vi "kalman predict step multi tick interval.vi"(7 "v-feedback":bool, 10 "state in":T1) -> (2 "state out":T1)   [LabVIEW 2010]
uses:
  integrating single axis kalman state.ctl
  <vilib>/rvi/FXPMathLib/FxpMul/XNode/nifxpmath_Multiplier.xnode
  <vilib>/rvi/FXPMathLib/FxpMul/subVIs/nifxpmath_Mul_SimConfig.ctl
  <vilib>/fxp/LVFixedPointQuantizationPolicyTypeDef.ctl
  <vilib>/fxp/LVFixedPointOverflowPolicyTypeDef.ctl
  <vilib>/rvi/FXPMathLib/FxpAdd/XNode/nifxpmath_Add.xnode
  <vilib>/rvi/FXPMathLib/FxpAdd/subVIs/nifxpmath_Add_SimConfig.ctl
  <vilib>/rvi/FXPMathLib/FxpInterpret/XNode/nifxpmath_Interpret.xnode
  <vilib>/rvi/FXPMathLib/FxpMul/simVIs/DllFxpMulTemp_sub.vi
  <vilib>/rvi/FXPMathLib/FxpAdd/simVIs/DllFxpAddTemp_sub.vi
panel:
  in  "elapsed time (ticks)":u32
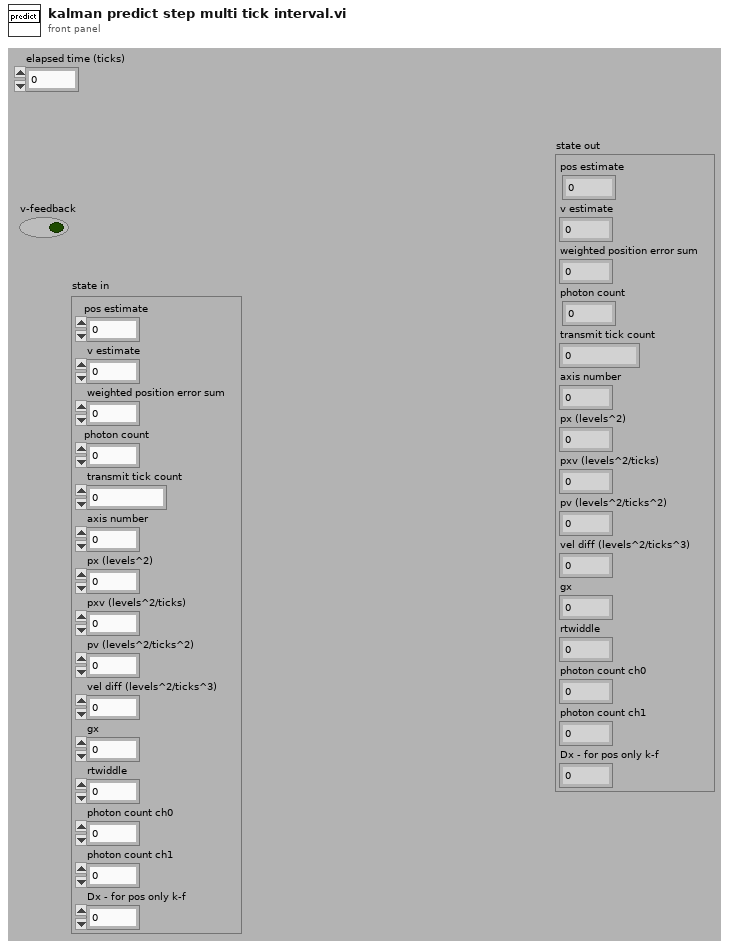
[diagram p1: front panel]
types:
  T1 = typedef "integrating single axis kalman state.ctl" = cluster{"pos estimate":fxp<+/-,32,16>, "v estimate":fxp<+/-,16,0>, "weighted position error sum":fxp<+/-,32,32>, "photon count":u32, "transmit tick count":u32, "axis number":u8, "px (levels^2)":fxp<+,32,19>, "pxv (levels^2/ticks)":fxp<+,32,2>, "pv (levels^2/ticks^2)":fxp<+,32,-14>, "vel diff (levels^2/ticks^3)":fxp<+,24,-22>, "gx":fxp<+,16,8>, "rtwiddle":fxp<+,16,26>, "photon count ch0":u32, "photon count ch1":u32, "Dx - for pos only k-f":fxp<+,32,19>}
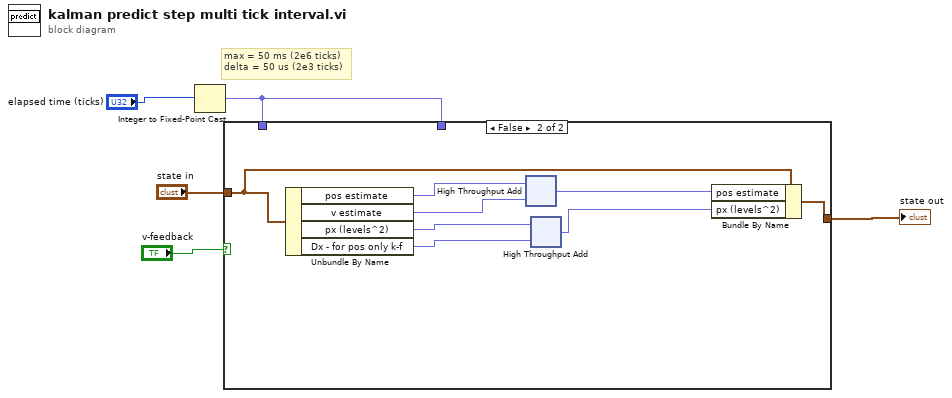
[diagram p0: block diagram]
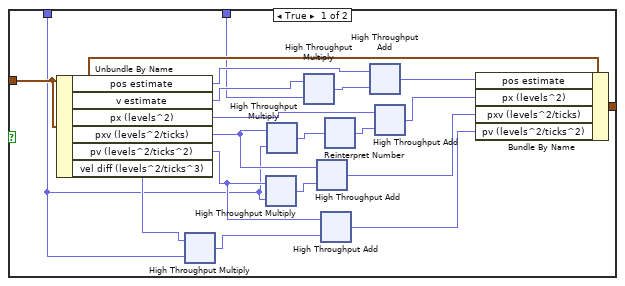
[diagram p2: hidden frame]
diagram:
  # "max = 50 ms (2e6 ticks)\ndelta = 50 us (2e3 ticks)"
  n1 = Integer to Fixed-Point Cast(integer="elapsed time (ticks)") -> (fixed-point=w1:fxp<+,10,21>)  [unwired: 1 in]
  n2 = case shown="False" "v-feedback" {
    tunnel: "state in" -> [w22 w275]
    tunnel: [w18 w273] -> w4
    tunnel: w1 -> [w14 _]
    tunnel: w1 -> [w7 _]
    frame True {
      n3 = Unbundle By Name(w22) -> ("pos estimate"=w17:fxp<+/-,32,16>, "v estimate"=w15:fxp<+/-,16,0>, "px (levels^2)"=w24:fxp<+,32,19>, "pxv (levels^2/ticks)"=w8:fxp<+,32,2>, "pv (levels^2/ticks^2)"=w10:fxp<+,32,-14>, "vel diff (levels^2/ticks^3)"=w12:fxp<+,24,-22>)
      n4 = xnode "High Throughput Multiply"("x"=w12, "y"=w7) -> ("x*y"=w11:fxp<+,16,-14>)
      n5 = xnode "High Throughput Multiply"("x"=w10, "y"=w7) -> ("x*y"=w9:fxp<+,16,2>)
      n6 = xnode "High Throughput Multiply"("x"=w8, "y"=w7) -> ("x*y"=w6:fxp<+,16,18>)
      n7 = xnode "High Throughput Multiply"("x"=w15, "y"=w14) -> ("x*y"=w13:fxp<+/-,16,15>)
      n8 = xnode "High Throughput Add"("x"=w8, "y"=w9) -> ("x+y"=w20:fxp<+,32,2>)
      n9 = xnode "High Throughput Add"("x"=w10, "y"=w11) -> ("x+y"=w19:fxp<+,32,-14>)
      n10 = xnode "Reinterpret Number"("x"=w6) -> ("y"=w23:fxp<+,16,19>)
      n11 = xnode "High Throughput Add"("x"=w17, "y"=w13) -> ("x+y"=w16:fxp<+/-,32,16>)
      n12 = xnode "High Throughput Add"("x"=w24, "y"=w23) -> ("x+y"=w21:fxp<+,32,19>)
      n13 = Bundle By Name(cluster=w22, "pos estimate"=w16, "px (levels^2)"=w21, "pxv (levels^2/ticks)"=w20, "pv (levels^2/ticks^2)"=w19) -> (w18:T1)
    }
    frame False {
      n14 = Unbundle By Name(w275) -> ("pos estimate"=w272:fxp<+/-,32,16>, "v estimate"=w277:fxp<+/-,16,0>, "px (levels^2)"=w276:fxp<+,32,19>, "Dx - for pos only k-f"=w270:fxp<+,32,19>)
      n15 = xnode "High Throughput Add"("x"=w272, "y"=w277) -> ("x+y"=w271:fxp<+/-,32,16>)
      n16 = xnode "High Throughput Add"("x"=w276, "y"=w270) -> ("x+y"=w274:fxp<+,32,19>)
      n17 = Bundle By Name(cluster=w275, "pos estimate"=w271, "px (levels^2)"=w274) -> (w273:T1)
    }
  }
  "state out" <- w4
